vi "PowerOn.vi"(0 "Universal Robot.lvclass in":refnum<class "Universal Robot.lvclass">, 5 "error in (no error)":errorcluster) -> (14 "Universal Robot.lvclass out":refnum<class "Universal Robot.lvclass">, 19 "error out":errorcluster)   [LabVIEW 2016, in "Universal Robot.lvclass"]
uses:
  Universal Robot.lvclass
  Universal Robot.lvclass/Universal Robot.ctl
  RobotMode.ctl
  Client Interfaces/Dashboard Server/Dashboard Server.lvclass
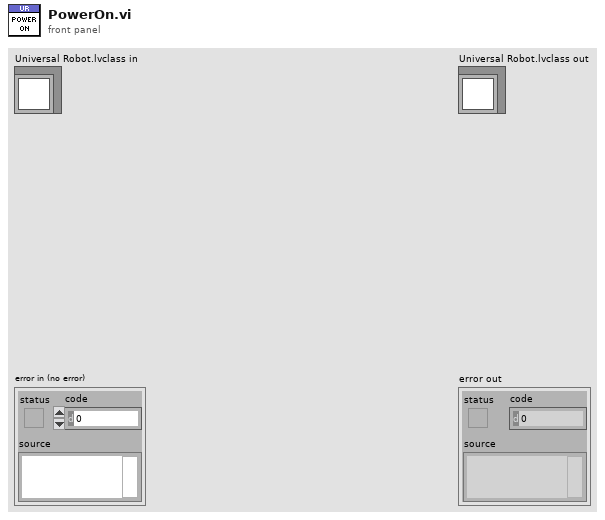
[diagram p1: front panel]
types:
  T1 = typedef "Universal Robot.lvclass/RobotMode.ctl" = enum16{"INVALID", "NO_CONTROLLER", "DISCONNECTED", "CONFIRM_SAFETY", "BOOTING", "POWER_OFF", "POWER_ON", "IDLE", "BACKDRIVE", "RUNNING"}
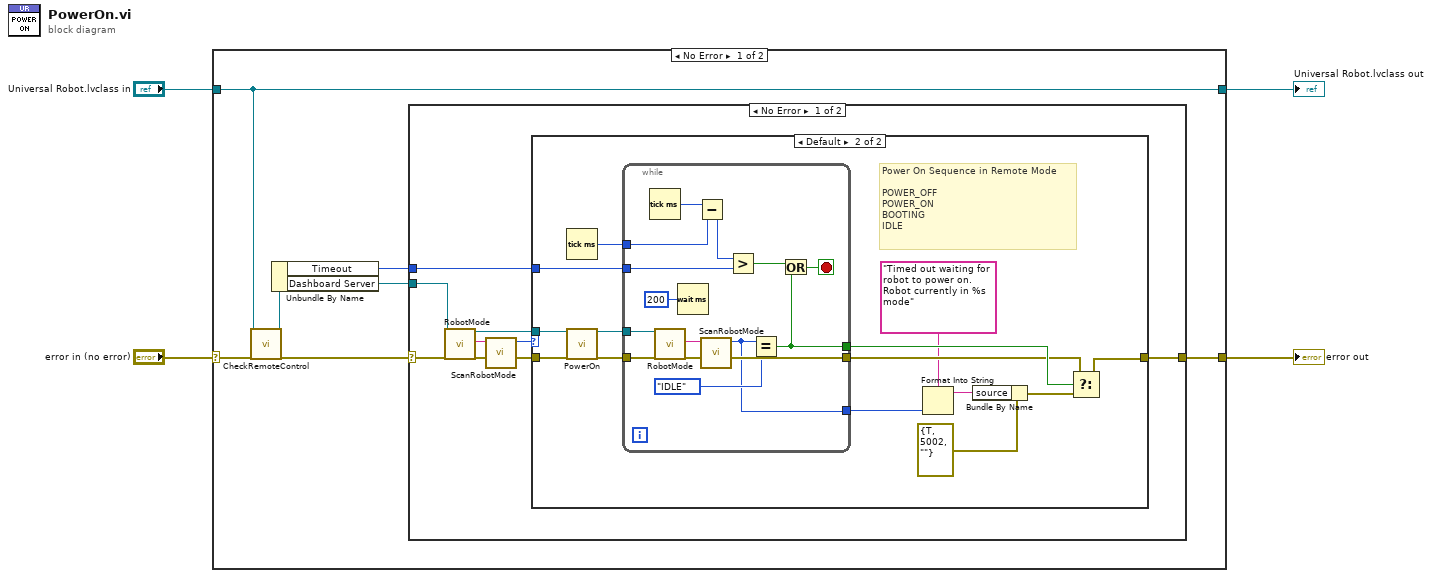
[diagram p0: block diagram]
diagram:
  n1 = case shown="No Error" "error in (no error)" {
    selector: "error in (no error)" -> [w10 w51]
    tunnel: [w11 w51] -> w3
    tunnel: "Universal Robot.lvclass in" -> [w9 w50]
    tunnel: [w9 w50] -> w1
    frame No Error {
      n2 = call-dynamic "CheckRemoteControl.vi"("Universal Robot.lvclass in"=w9, "error in (no error)"=w10) -> ("Universal Robot.lvclass out"=w8:refnum<class "Universal Robot.lvclass">, "error out"=w5:errorcluster)  [unwired: 16 in]
      n3 = Unbundle By Name(w8) -> ("Timeout"=w6:u32, "Dashboard Server"=w7:refnum<class "Dashboard Server.lvclass">)
      n4 = case shown="No Error" w5 {
        selector: w5 -> [w14 w49]
        tunnel: [w19 w49] -> w11
        tunnel: w7 -> [w18 _]
        tunnel: w6 -> [w17 _]
        frame No Error {
          n5 = call-dynamic "RobotMode.vi"("DashboardServer in"=w18, "error in (no error)"=w14) -> ("DashboardServer out"=w15:refnum<class "Dashboard Server.lvclass">, "robotMode"=w13:string, "error out"=w16:errorcluster)  [unwired: 15 in]
          n6 = call "ScanRobotMode.vi"("robotMode in"=w13) -> ("robotMode out"=w12:T1)  [unwired: 10 in]
          n7 = case shown="Default" w12 {
            tunnel: [w20 w26] -> w19
            tunnel: w16 -> [w20 w32]
            tunnel: w15 -> [_ w31]
            tunnel: w17 -> [_ w30]
            frame "RUNNING" {
              # "Robot is already running"
            }
            frame Default {
              # "Power On Sequence in Remote Mode\n\nPOWER_OFF\nPOWER_ON\nBOOTING\nIDLE"
              n8 = Tick Count (ms)() -> (millisecond timer value=w29:u32)
              n9 = call-dynamic "PowerOn.vi"("DashboardServer in"=w31, "error in (no error)"=w32) -> ("DashboardServer out"=w33:refnum<class "Dashboard Server.lvclass">, "error out"=w34:errorcluster)  [unwired: 15 in, 1 out]
              n10 = while {
                tunnel: w33 -> [w47]
                tunnel: w34 -> [w48]
                tunnel: [w46] -> w27
                tunnel: w30 -> [w44]
                tunnel: w29 -> [w43]
                tunnel: [w38] -> w28
                tunnel: [w35] -> w25
                stop <- w39 stop-if-true
                n11 = Tick Count (ms)() -> (millisecond timer value=w42:u32)
                n12 = call-dynamic "RobotMode.vi"("DashboardServer in"=w47, "error in (no error)"=w48) -> ("robotMode"=w37:string, "error out"=w46:errorcluster)  [unwired: 15 in, 1 out]
                n13 = Wait (ms)(milliseconds to wait=u32 200) -> ()  [unwired: 1 out]
                n14 = Subtract(x=w42, y=w43) -> (x-y=w41:u32)
                n15 = call "ScanRobotMode.vi"("robotMode in"=w37) -> ("robotMode out"=w35:T1)  [unwired: 10 in]
                n16 = Greater?(x=w41, y=w44) -> (0:w40:bool)
                n17 = Equal?(x=w35, y=RobotMode."IDLE") -> (x = y?=w38:bool)
                n18 = Or(x=w40, y=w38) -> (x .or. y?=w39:bool)
              }
              n19 = Format Into String(format string="Timed out waiting for robot to power on. Robot currently in %s mode", w25) -> (resulting string=w23:string)  [unwired: 2 in, 1 out]
              n20 = Bundle By Name(cluster=errorcluster {"status"=TRUE, "code"=5002, "source"=""} ("error constant"), "source"=w23) -> (w22:errorcluster)
              n21 = Select(t=w27, s=w28, f=w22) -> (s? t:f=w26:errorcluster)
            }
          }
        }
        frame Error {
        }
      }
    }
    frame Error {
    }
  }
  "error out" <- w3
  "Universal Robot.lvclass out" <- w1
